vi "Read Dashboard Variables.vi"() -> ()   [LabVIEW 2020]
uses:
  <vilib>/Rock Robotics/Network Tables/NT Read Number.vi
  Framework/Robot Global Data.vi
  <vilib>/Rock Robotics/Network Tables/NT Read String.vi
panel:
  out "Shooter Auto Setpoint":dbl=0.8 format="%#_13g"
  out "MaxDrive":dbl(slide)=0.6824817518248175 min=0.0 max=1.0 step=0.01 scale=0.0..1.0
  out "DriveK":dbl(slide)=0.26277372262773724 min=0.0 max=1.0 step=0.05 scale=0.0..1.0
  out "Limelight Goal Area":dbl(slide)=14.8723 min=0.1 max=25.0 step=0.25 scale=0.0..25.0
  out "AimDeadband":dbl min=0.0 max=10.0 step=0.25
  out "MinSteerCommand":dbl(slide)=0.2717391304347826 min=0.0 max=0.5 step=0.05 scale=0.0..0.5
  out "SteeringK":dbl(slide)=0.025362318840579712 min=0.0 max=0.25 step=0.01 scale=0.0..0.25
  out "Shooter Setpoint Reverse":dbl=0.8 format="%#_13g"
  out "Transfer Release Setpoint Reverse":dbl
  out "Intake Reverse Setpoint":dbl=0.8 format="%#_13g"
  out "Reverse Duration":dbl=3.0 format="%#_13g"
  out "Intake Sped Up Setpoint":dbl=0.8 format="%#_13g"
  out "Intake Sped Up Duration":dbl=3.0 format="%#_13g"
  out "Custom MaxSpeedSlow (0.6)":dbl=0.6
  out "Transfer Release Duration":dbl
  out "Transfer Up Duration":dbl
  out "Pivot Duration":dbl
  out "Pivot Right Speed":dbl
  out "Pivot Left Speed":dbl
  out "Transfer Release Setpoint":dbl
  out "Transfer Up Setpoint":dbl
  out "Intake Setpoint":dbl=0.8 format="%#_13g"
  out "Intake Duration (s)":dbl=3.0 format="%#_13g"
  out "Shooter Duration":dbl=3.0 format="%#_13g"
  out "Shooter Setpoint":dbl=0.8 format="%#_13g"
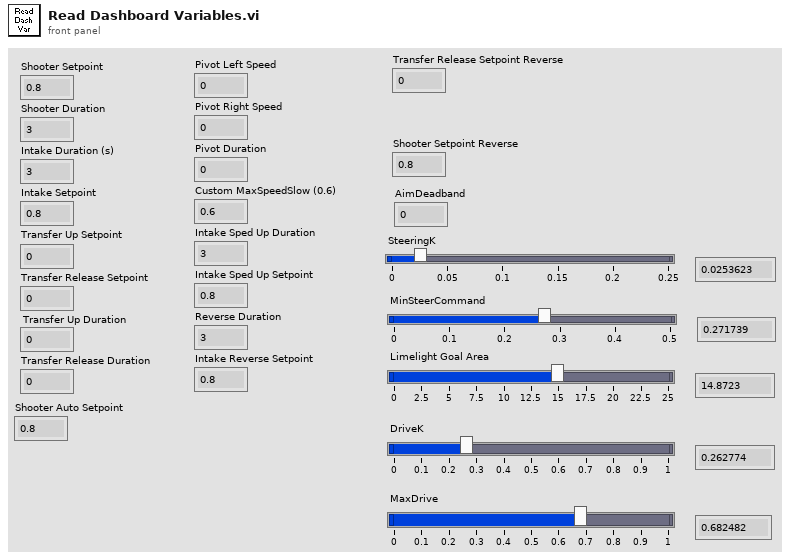
[diagram p1: front panel]
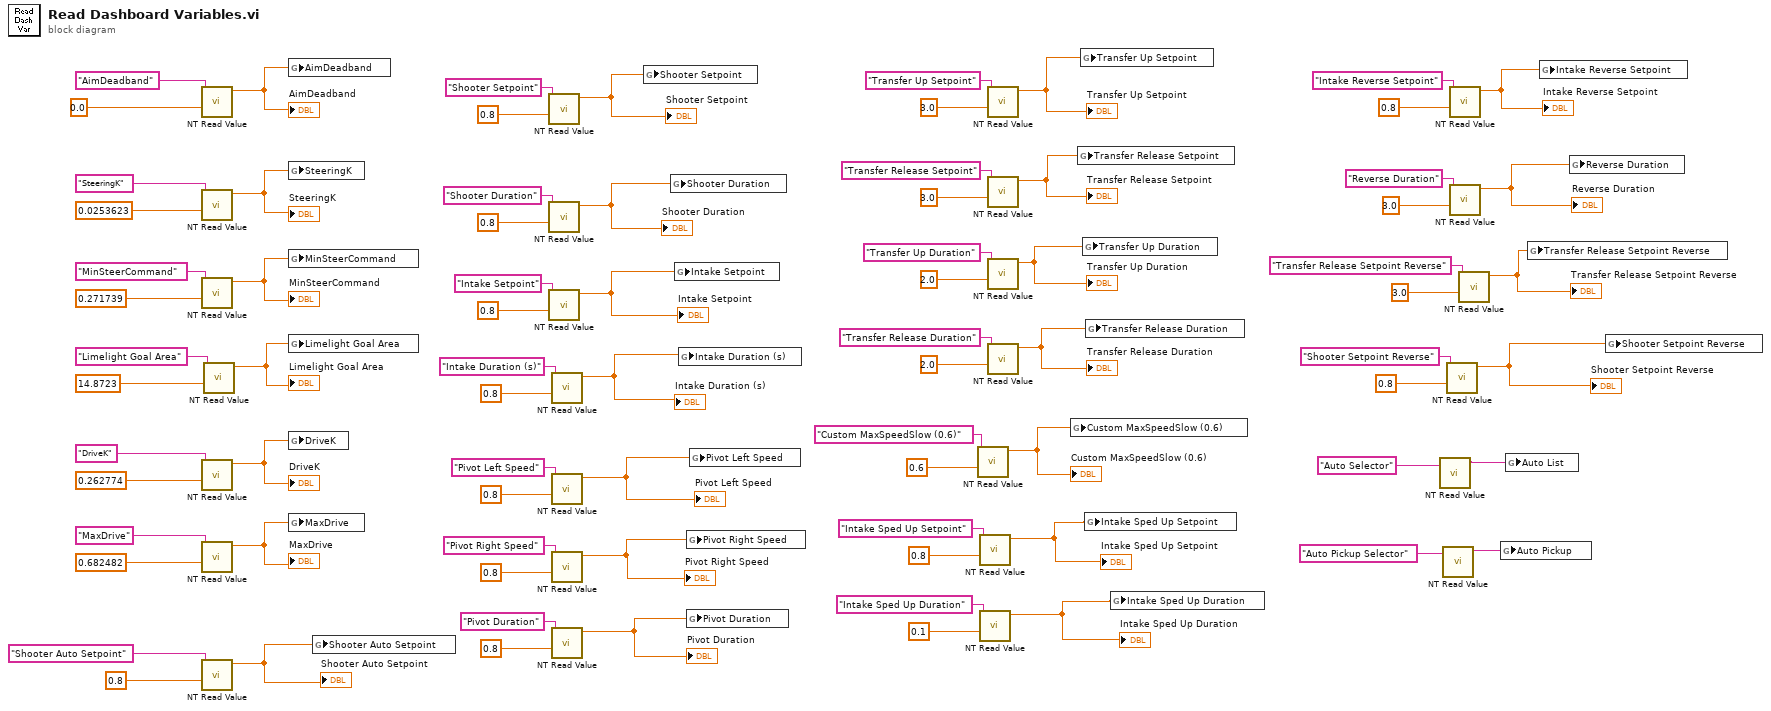
[diagram p0: block diagram]
diagram:
  n1 = call-poly <vilib>:"NT Read Value.vi"("Default Value"=0.0, "Name"="AimDeadband") -> ("Numeric"=w9:dbl)  [unwired: 8 in, 1 out]
  "AimDeadband" <- w9
  n2 = call-poly <vilib>:"NT Read Value.vi"("Default Value"=0.0253623, "Name"="SteeringK") -> ("Numeric"=w8:dbl)  [unwired: 8 in, 1 out]
  "SteeringK" <- w8
  n3 = call-poly <vilib>:"NT Read Value.vi"("Default Value"=0.271739, "Name"="MinSteerCommand") -> ("Numeric"=w7:dbl)  [unwired: 8 in, 1 out]
  "MinSteerCommand" <- w7
  n4 = call-poly <vilib>:"NT Read Value.vi"("Default Value"=0.262774, "Name"="DriveK") -> ("Numeric"=w5:dbl)  [unwired: 8 in, 1 out]
  "DriveK" <- w5
  n5 = call-poly <vilib>:"NT Read Value.vi"("Default Value"=0.682482, "Name"="MaxDrive") -> ("Numeric"=w4:dbl)  [unwired: 8 in, 1 out]
  "MaxDrive" <- w4
  n6 = call-poly <vilib>:"NT Read Value.vi"("Default Value"=0.8, "Name"="Shooter Auto Setpoint") -> ("Numeric"=w1:dbl)  [unwired: 8 in, 1 out]
  "Shooter Auto Setpoint" <- w1
  n7 = call-poly <vilib>:"NT Read Value.vi"("Default Value"=14.8723, "Name"="Limelight Goal Area") -> ("Numeric"=w6:dbl)  [unwired: 8 in, 1 out]
  "Limelight Goal Area" <- w6
  n8 = global write "Robot Global Data.vi" "AimDeadband"(w9) -> ()
  n9 = global write "Robot Global Data.vi" "SteeringK"(w8) -> ()
  n10 = global write "Robot Global Data.vi" "MinSteerCommand"(w7) -> ()
  n11 = global write "Robot Global Data.vi" "Limelight Goal Area"(w6) -> ()
  n12 = global write "Robot Global Data.vi" "DriveK"(w5) -> ()
  n13 = global write "Robot Global Data.vi" "MaxDrive"(w4) -> ()
  n14 = global write "Robot Global Data.vi" "Shooter Auto Setpoint"(w1) -> ()
  n15 = call-poly <vilib>:"NT Read Value.vi"("Default Value"=0.8, "Name"="Shooter Setpoint") -> ("Numeric"=w77:dbl)  [unwired: 8 in, 1 out]
  "Shooter Setpoint" <- w77
  n16 = call-poly <vilib>:"NT Read Value.vi"("Default Value"=0.8, "Name"="Shooter Duration") -> ("Numeric"=w74:dbl)  [unwired: 8 in, 1 out]
  "Shooter Duration" <- w74
  n17 = call-poly <vilib>:"NT Read Value.vi"("Default Value"=0.8, "Name"="Intake Setpoint") -> ("Numeric"=w69:dbl)  [unwired: 8 in, 1 out]
  "Intake Setpoint" <- w69
  n18 = call-poly <vilib>:"NT Read Value.vi"("Default Value"=0.8, "Name"="Intake Duration (s)") -> ("Numeric"=w68:dbl)  [unwired: 8 in, 1 out]
  "Intake Duration (s)" <- w68
  n19 = call-poly <vilib>:"NT Read Value.vi"("Default Value"=0.8, "Name"="Pivot Left Speed") -> ("Numeric"=w57:dbl)  [unwired: 8 in, 1 out]
  "Pivot Left Speed" <- w57
  n20 = call-poly <vilib>:"NT Read Value.vi"("Default Value"=0.8, "Name"="Pivot Right Speed") -> ("Numeric"=w58:dbl)  [unwired: 8 in, 1 out]
  "Pivot Right Speed" <- w58
  n21 = call-poly <vilib>:"NT Read Value.vi"("Default Value"=0.8, "Name"="Pivot Duration") -> ("Numeric"=w59:dbl)  [unwired: 8 in, 1 out]
  "Pivot Duration" <- w59
  n22 = global write "Robot Global Data.vi" "Shooter Setpoint"(w77) -> ()
  n23 = global write "Robot Global Data.vi" "Shooter Duration"(w74) -> ()
  n24 = global write "Robot Global Data.vi" "Intake Setpoint"(w69) -> ()
  n25 = global write "Robot Global Data.vi" "Intake Duration (s)"(w68) -> ()
  n26 = global write "Robot Global Data.vi" "Pivot Right Speed"(w58) -> ()
  n27 = global write "Robot Global Data.vi" "Pivot Duration"(w59) -> ()
  n28 = global write "Robot Global Data.vi" "Pivot Left Speed"(w57) -> ()
  n29 = call-poly <vilib>:"NT Read Value.vi"("Default Value"=0.6, "Name"="Custom MaxSpeedSlow (0.6)") -> ("Numeric"=w40:dbl)  [unwired: 8 in, 1 out]
  "Custom MaxSpeedSlow (0.6)" <- w40
  n30 = call-poly <vilib>:"NT Read Value.vi"("Default Value"=0.8, "Name"="Intake Sped Up Setpoint") -> ("Numeric"=w35:dbl)  [unwired: 8 in, 1 out]
  "Intake Sped Up Setpoint" <- w35
  n31 = call-poly <vilib>:"NT Read Value.vi"("Default Value"=0.1, "Name"="Intake Sped Up Duration") -> ("Numeric"=w34:dbl)  [unwired: 8 in, 1 out]
  "Intake Sped Up Duration" <- w34
  n32 = call-poly <vilib>:"NT Read Value.vi"("Default Value"=3.0, "Name"="Transfer Up Setpoint") -> ("Numeric"=w50:dbl)  [unwired: 8 in, 1 out]
  "Transfer Up Setpoint" <- w50
  n33 = call-poly <vilib>:"NT Read Value.vi"("Default Value"=3.0, "Name"="Transfer Release Setpoint") -> ("Numeric"=w49:dbl)  [unwired: 8 in, 1 out]
  "Transfer Release Setpoint" <- w49
  n34 = call-poly <vilib>:"NT Read Value.vi"("Default Value"=2.0, "Name"="Transfer Up Duration") -> ("Numeric"=w47:dbl)  [unwired: 8 in, 1 out]
  "Transfer Up Duration" <- w47
  n35 = call-poly <vilib>:"NT Read Value.vi"("Default Value"=2.0, "Name"="Transfer Release Duration") -> ("Numeric"=w48:dbl)  [unwired: 8 in, 1 out]
  "Transfer Release Duration" <- w48
  n36 = global write "Robot Global Data.vi" "Custom MaxSpeedSlow (0.6)"(w40) -> ()
  n37 = global write "Robot Global Data.vi" "Transfer Release Setpoint"(w49) -> ()
  n38 = global write "Robot Global Data.vi" "Transfer Up Setpoint"(w50) -> ()
  n39 = global write "Robot Global Data.vi" "Transfer Up Duration"(w47) -> ()
  n40 = global write "Robot Global Data.vi" "Intake Sped Up Setpoint"(w35) -> ()
  n41 = global write "Robot Global Data.vi" "Transfer Release Duration"(w48) -> ()
  n42 = global write "Robot Global Data.vi" "Intake Sped Up Duration"(w34) -> ()
  n43 = call-poly <vilib>:"NT Read Value.vi"("Name"="Auto Selector") -> ("String"=w44:string)  [unwired: 9 in, 1 out]
  n44 = call-poly <vilib>:"NT Read Value.vi"("Name"="Auto Pickup Selector") -> ("String"=w43:string)  [unwired: 9 in, 1 out]
  n45 = call-poly <vilib>:"NT Read Value.vi"("Default Value"=0.8, "Name"="Shooter Setpoint Reverse") -> ("Numeric"=w22:dbl)  [unwired: 8 in, 1 out]
  "Shooter Setpoint Reverse" <- w22
  n46 = call-poly <vilib>:"NT Read Value.vi"("Default Value"=0.8, "Name"="Intake Reverse Setpoint") -> ("Numeric"=w28:dbl)  [unwired: 8 in, 1 out]
  "Intake Reverse Setpoint" <- w28
  n47 = call-poly <vilib>:"NT Read Value.vi"("Default Value"=3.0, "Name"="Reverse Duration") -> ("Numeric"=w29:dbl)  [unwired: 8 in, 1 out]
  "Reverse Duration" <- w29
  n48 = call-poly <vilib>:"NT Read Value.vi"("Default Value"=3.0, "Name"="Transfer Release Setpoint Reverse") -> ("Numeric"=w25:dbl)  [unwired: 8 in, 1 out]
  "Transfer Release Setpoint Reverse" <- w25
  n49 = global write "Robot Global Data.vi" "Auto Pickup"(w43) -> ()
  n50 = global write "Robot Global Data.vi" "Auto List"(w44) -> ()
  n51 = global write "Robot Global Data.vi" "Transfer Release Setpoint Reverse"(w25) -> ()
  n52 = global write "Robot Global Data.vi" "Intake Reverse Setpoint"(w28) -> ()
  n53 = global write "Robot Global Data.vi" "Reverse Duration"(w29) -> ()
  n54 = global write "Robot Global Data.vi" "Shooter Setpoint Reverse"(w22) -> ()
